vi "SG_NetworkListener.vi"(8 "error in (no error)":errorcluster, 10 "time-out":i32, 11 "Gserver in":refnum<class "Gserver.lvclass">) -> (0 "error out":errorcluster, 3 "Gserver out":refnum<class "Gserver.lvclass">)   [LabVIEW 2020, in "Sgraph_lib_V1.lvlib" / "Gserver.lvclass"]
doc: "Andre Koelewijn, 24 June 2023\n\nSgraph Network Listener.\nWaits for a new network connection that can be used to remotely query the Sgraph historian"
uses:
  Gserver.lvclass
  Gserver.lvclass/Gserver.ctl
  controls/SG_NetworkClient.ctl
  controls/Typedef_Gviewer-Query.ctl
  controls/Typedef_QueryType.ctl
  Builds/Sgraph_lib_V1.lvlib
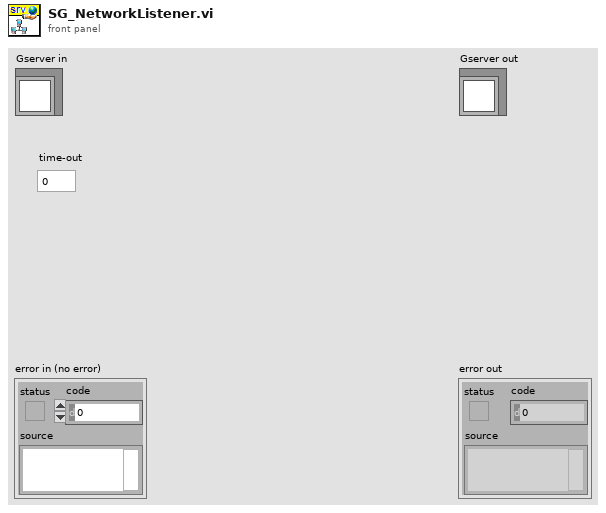
[diagram p1: front panel]
types:
  T1 = typedef "Sgraph_lib_V1.lvlib/Gserver.lvclass/SG_NetworkClient.ctl" = cluster{"address":string, "port":u16, "connection-ID":refnum<k5>}
  T2 = typedef "Sgraph_lib_V1.lvlib/Gserver.lvclass/Typedef_QueryType.ctl" = enum16{"Subscribe", "SubscribeNetw", "DataRequest", "RequestAllTags", "RequestIniPath", "FAMMstarted", "SetClientOptions", "GviewerUpdate", "OpenNewGraph", "CloseClient", "CloseAllClients", "Close Gserver", "OpenMemoryMap", "MeMapDataRequest", "MeMapDataResponse", "OpenDBeditor", "CheckDBeditorRunning", "StoppedDBeditor", "SaveDB_TAGpropRecord", "ConfirmDB_TAGpropSave", "GetXconstraints", "OpenNewNetworkGraph"}
  T3 = typedef "Sgraph_lib_V1.lvlib/Gserver.lvclass/Typedef_Gviewer-Query.ctl" = cluster{"Query_type":T2, "data":variant, "Source":string, "Time Stamp":timestamp}
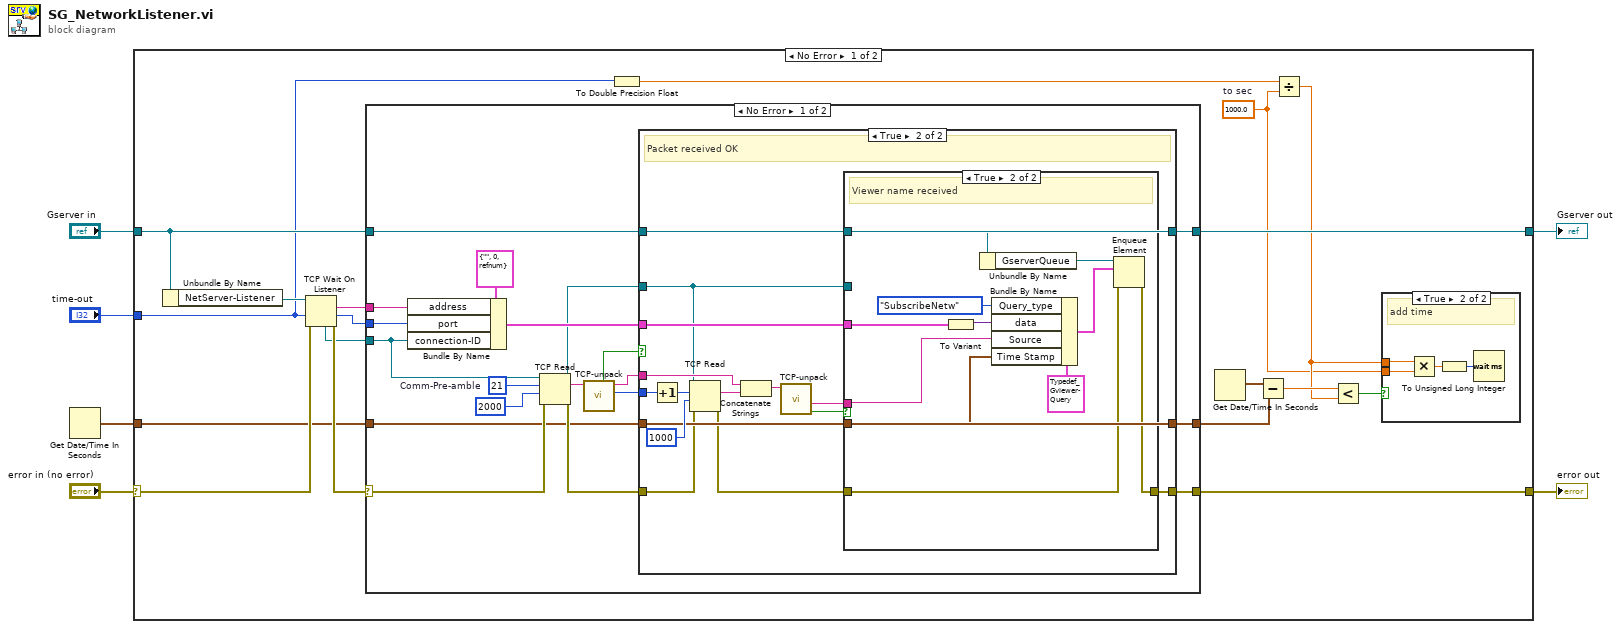
[diagram p0: block diagram]
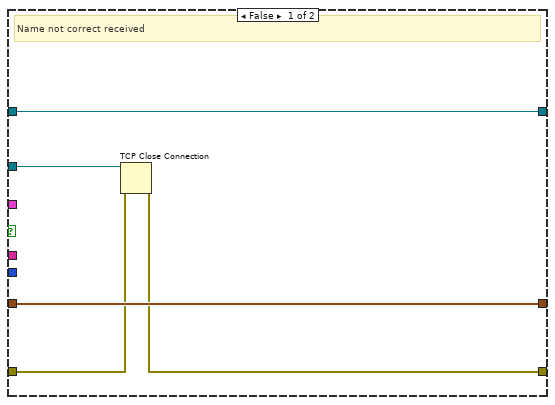
[diagram p3: hidden frame]
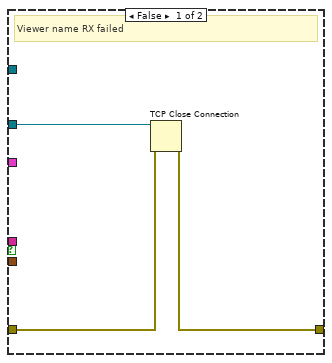
[diagram p4: hidden frame]
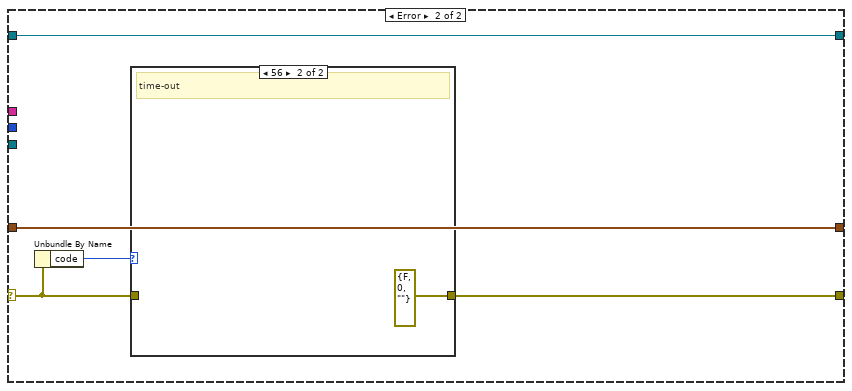
[diagram p5: hidden frame]
diagram:
  n1 = Get Date/Time In Seconds() -> (seconds since 1Jan1904=w1:timestamp)
  n2 = case shown="No Error" "error in (no error)" {
    selector: "error in (no error)" -> [w23 w90]
    tunnel: [w21 w90] -> w5
    tunnel: [w19 w89] -> w3
    tunnel: "Gserver in" -> [w20 w89]
    tunnel: "time-out" -> [w12 _]
    tunnel: w1 -> [w15 _]
    frame No Error {
      w7 = 1000.0  # to sec
      n3 = Unbundle By Name(w20) -> ("NetServer-Listener"=w24:refnum<k5>)
      n4 = TCP Wait On Listener(8:w23, 9:w12, 11:w24) -> (0:w22:errorcluster, 1:w17:u16, 2:w18:string, 4:w16:refnum<k5>)  [unwired: 1 in, 1 out]
      n5 = case shown="No Error" w22 {
        selector: w22 -> [w39 w83]
        tunnel: [w43 w82] -> w21
        tunnel: w20 -> [w44 w86]
        tunnel: [w33 w86] -> w19
        tunnel: w18 -> [w46 _]
        tunnel: w17 -> [w45 _]
        tunnel: w16 -> [w41 _]
        tunnel: w15 -> [w35 w85]
        tunnel: [w34 w85] -> w13
        frame No Error {
          w40 = 21  # Comm-Pre-amble
          n6 = Bundle By Name(cluster=T1 {"address"="", "port"=0, "connection-ID"=refnum} ("SG_Client"), "address"=w46, "port"=w45, "connection-ID"=w41) -> (w42:T1)
          n7 = TCP Read(connection ID=w41, bytes to read=w40, error in (no error)=w39, 9:2000 ("timeout ms (25000)")) -> (connection ID out=w32:refnum<k5>, data out=w36:string, error out=w38:errorcluster)  [unwired: 1 in]
          n8 = call "TCP-unpack.vi"("TCP RX in"=w36) -> ("bytecount"=w29:i32, "TCP RX out (rest)"=w31:string, "CountOK"=w30:bool)  [unwired: 6 in, 2 out]
          n9 = case shown="True" w30 {
            tunnel: w44 -> [w51 w65]
            tunnel: [w49 w67] -> w43
            tunnel: w42 -> [_ w66]
            tunnel: w38 -> [w48 w60]
            tunnel: w35 -> [w52 w62]
            tunnel: [w52 w62] -> w34
            tunnel: [w51 w65] -> w33
            tunnel: w32 -> [w50 w54]
            tunnel: w31 -> [_ w58]
            tunnel: w29 -> [_ w64]
            frame False {
              # "Name not correct received"
              n10 = TCP Close Connection(connection ID=w50, error in (no error)=w48) -> (error out=w49:errorcluster)  [unwired: 1 in, 1 out]
            }
            frame True {
              # "Packet received OK"
              n11 = Increment(x=w64) -> (x+1=w53:i32)
              n12 = TCP Read(connection ID=w54, bytes to read=w53, error in (no error)=w60, 9:1000 ("timeout ms (25000)")) -> (data out=w59:string, error out=w61:errorcluster)  [unwired: 1 in, 1 out]
              n13 = Concatenate Strings(w58, w59) -> (w57:string)
              n14 = call "TCP-unpack.vi"("TCP RX in"=w57) -> ("Success"=w56:bool, "TCP data"=w55:string)  [unwired: 6 in, 3 out]
              n15 = case shown="True" w56 {
                tunnel: [w68 w80] -> w67
                tunnel: w66 -> [_ w76]
                tunnel: w65 -> [_ w74]
                tunnel: w62 -> [_ w73]
                tunnel: w61 -> [w69 w72]
                tunnel: w55 -> [_ w71]
                tunnel: w54 -> [w70 _]
                frame False {
                  # "Viewer name RX failed"
                  n16 = TCP Close Connection(connection ID=w70, error in (no error)=w69) -> (error out=w68:errorcluster)  [unwired: 1 in, 1 out]
                }
                frame True {
                  # "Viewer name received"
                  n17 = To Variant(anything=w76) -> (Variant=w75:variant)
                  n18 = Unbundle By Name(w74) -> ("GserverQueue"=w81:refnum<queue>)
                  n19 = Bundle By Name(cluster=T3 {"Query_type"=enum."Subscribe", "data"=variant, "Source"="", "Time Stamp"=timestamp(0 s since 1904-01-01)} ("element"), "Query_type"=Typedef_QueryType."SubscribeNetw", "data"=w75, "Source"=w71, "Time Stamp"=w73) -> (w78:T3)
                  n20 = Enqueue Element(queue=w81, element=w78, error in (no error)=w72) -> (error out=w80:errorcluster)  [unwired: 1 in, 2 out]
                }
              }
            }
          }
        }
        frame Error {
          n21 = Unbundle By Name(w83) -> ("code"=w84:i32)
          n22 = case shown="56" w84 {
            tunnel: w83 -> [w87 _]
            tunnel: [w87 errorcluster {"status"=FALSE, "code"=0, "source"=""} ("error IO")] -> w82
            frame Default {
              # "no time-out"
            }
            frame 56 {
              # "time-out"
            }
          }
        }
      }
      n23 = To Double Precision Float(number=w12) -> (double precision float=w10:dbl)
      n24 = Get Date/Time In Seconds() -> (seconds since 1Jan1904=w14:timestamp)
      n25 = Subtract(x=w14, y=w13) -> (x-y=w11:dbl)
      n26 = Divide(x=w10, y=w7) -> (x/y=w8:dbl)
      n27 = Less?(x=w11, y=w8) -> (x < y?=w9:bool)
      n28 = case shown="True" w9 {
        tunnel: w8 -> [_ w28]
        tunnel: w7 -> [_ w27]
        frame False {
        }
        frame True {
          # "add time"
          n29 = Multiply(x=w28, y=w27) -> (x*y=w26:dbl)
          n30 = To Unsigned Long Integer(number=w26) -> (unsigned 32bit integer=w25:u32)
          n31 = Wait (ms)(milliseconds to wait=w25) -> ()  [unwired: 1 out]
        }
      }
    }
    frame Error {
    }
  }
  "error out" <- w5
  "Gserver out" <- w3
